vi "command engine process responses.vi"(8 "error out":errorcluster, 9 "State Variables":T1, 10 "Parameters":T4 {"Compiled"."MetaData"."Refs"."Data Reference" format="%.0x"; "Compiled"."Triggers"."Chan Refs" format="%.0x"; "Compiled"."Statuses"."Refs" format="%.0x"; "Compiled"."Data"."Refs" format="%.0x"; "Compiled"."Periodic Enable"."Refs"."Data Reference" format="%.0x"; "Compiled"."Wait Values"."Refs"."Data Reference" format="%.0x"; "Compiled"."External Channels"."Channels" format="%.0x"; "Compiled"."External Channels"."Triggers" format="%.0x"}, 11 "Global Variables":T17) -> (0 "error out":errorcluster, 1 "State Variables out":T1, 2 "Parameters out":T4 {"Compiled"."MetaData"."Refs"."Data Reference" format="%.0x"; "Compiled"."Triggers"."Chan Refs" format="%.0x"; "Compiled"."Statuses"."Refs" format="%.0x"; "Compiled"."Data"."Refs" format="%.0x"; "Compiled"."Periodic Enable"."Refs"."Data Reference" format="%.0x"; "Compiled"."Wait Values"."Refs"."Data Reference" format="%.0x"; "Compiled"."External Channels"."Channels" format="%.0x"; "Compiled"."External Channels"."Triggers" format="%.0x"}, 3 "Global Variables out":T17)   [LabVIEW 2013, in "Instrument Addon Engine.lvlib"]
uses:
  Instrument Addon Engine.lvlib
  Inline Async API/Controls/Engine State Variables.ctl
  Network Communication/TCP Refs.ctl
  Network Communication/Network Comm Global Ref.ctl
  Stop FG/Stop Global Ref.ctl
  <vilib>/NI/AMC/Message Queue.ctl
  <vilib>/NI/AMC/Message.ctl
  <vilib>/NI/Tools/Keyed Array/KeyedArray.ctl
  Types/Commands RT Configuration Cluster.ctl
  Protocols.lvlibp/Protocol Parent/Protocol Parent.lvclass
  Shared/Types/Compiled Settings.ctl
  Shared/Types/Command Parameters.ctl
  Shared/Types/Linked Channel Cluster.ctl
  <vilib>/NI Veristand/Custom Device API/Block Data Reference.ctl
  <vilib>/NI Veristand/Custom Device API/Data Reference.ctl
  Shared/Types/Response RT Configuration Cluster.ctl
  Shared/Types/Response Parameters.ctl
  Shared/Types/Response Wait Type.ctl
  Shared/Types/Message Parameters.ctl
  Shared/Types/Message Generation Type.ctl
  Shared/Types/External Trigger Refs.ctl
  Types/FIFO References.ctl
  Protections.lvlibp/Parent Protection/Protection.lvclass
  command engine global variables.ctl
  Stop FG/Stop FG.lvlib
  Network Communication/Network Common API.lvlib
  <vilib>/NI/Tools/Keyed Array/Tools_KeyedArray.lvlib
  <vilib>/NI/AMC/AMC.lvlib
  Inline Async API/Inline Async API.lvlib
  Shared/Instrument Addon Shared.lvlib
  <vilib>/NI Veristand/Custom Device API/Custom Device API.lvlib
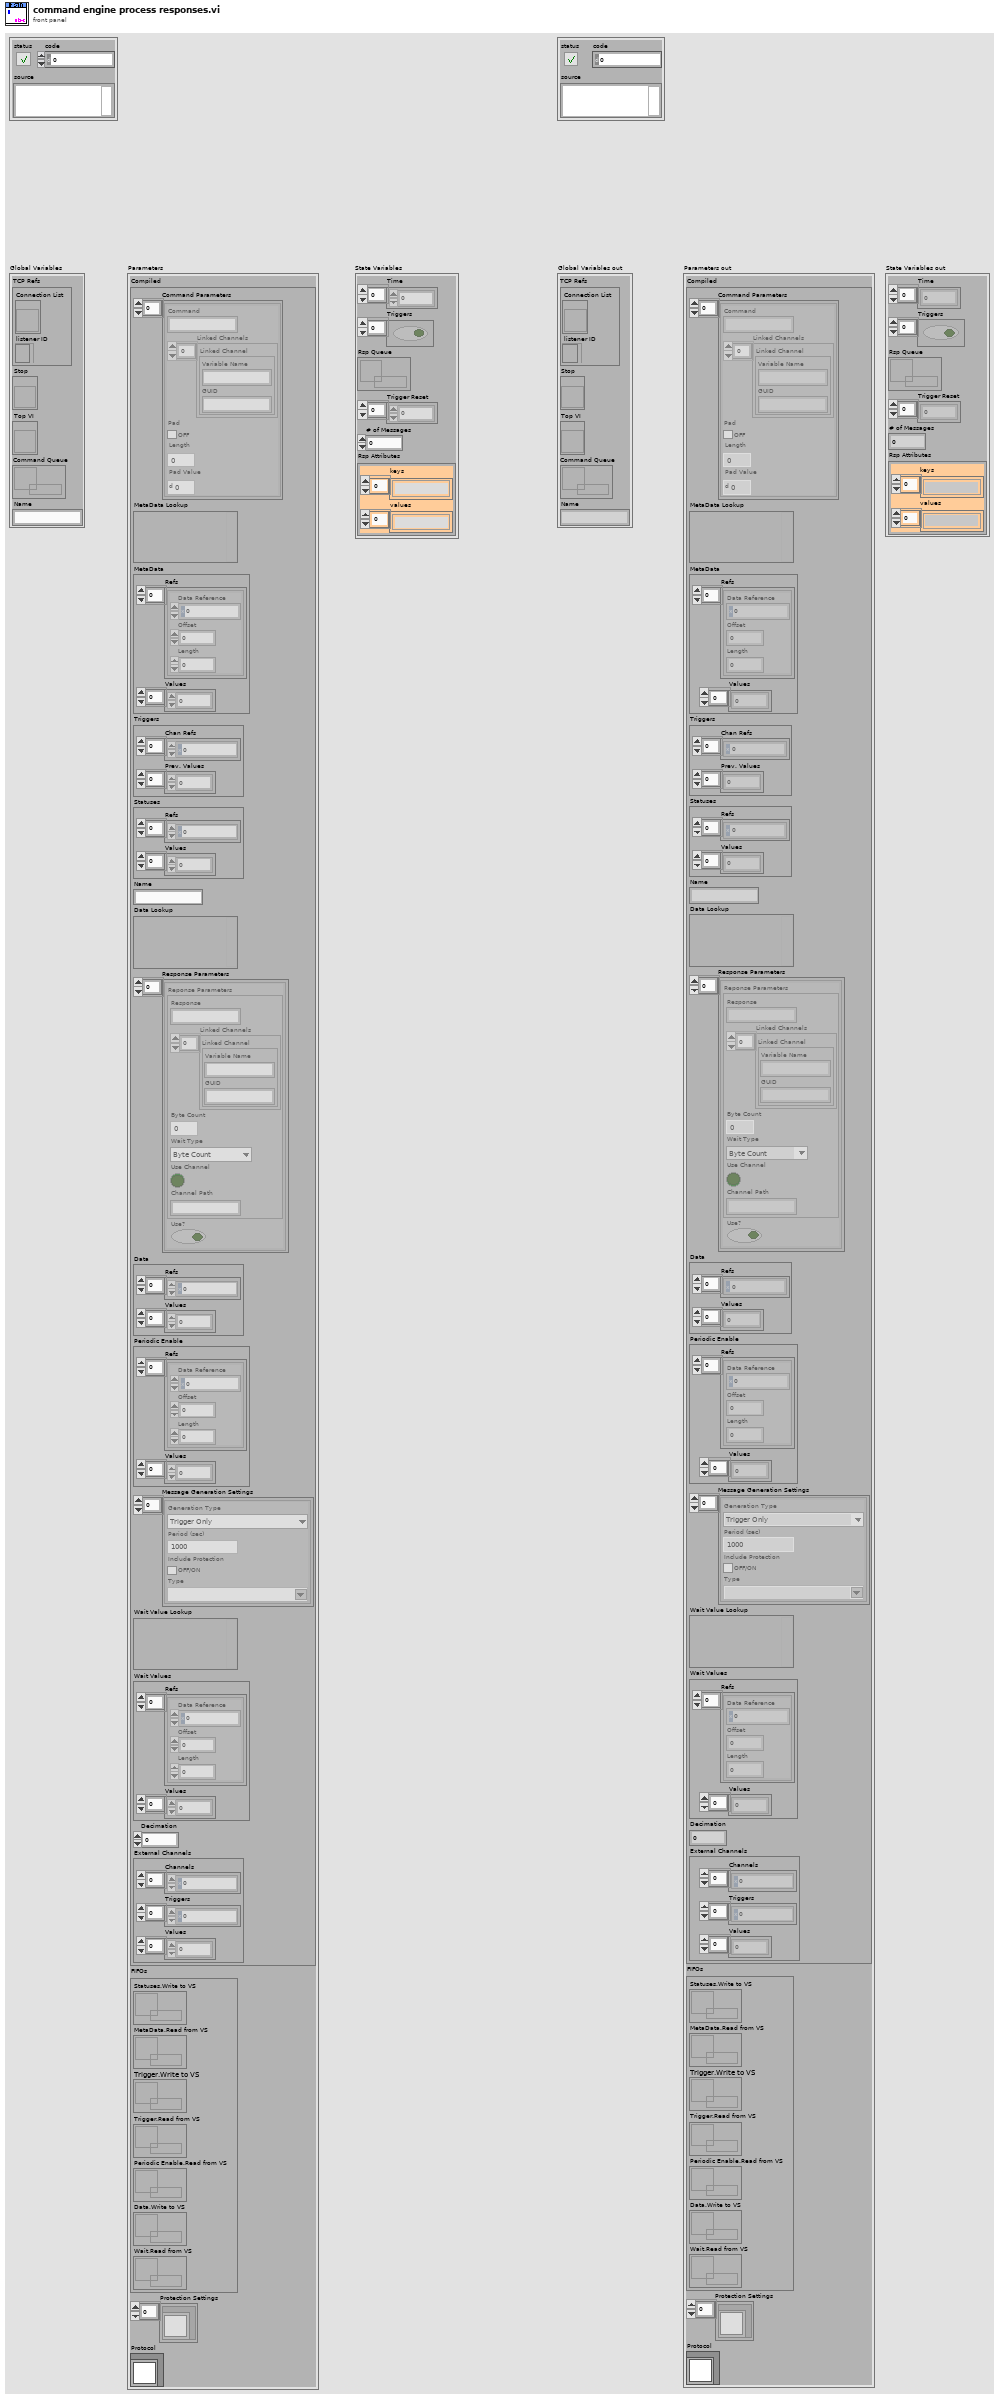
[diagram p1: front panel]
types:
  T1 = typedef "Instrument Addon Engine.lvlib/command engine global variables.ctl" = cluster{"Time":u32[], "Triggers":bool[], "Rsp Queue":T2, "Trigger Reset":dbl[], "# of Messages":i32, "Rsp Attributes":T3}
  T2 = typedef "AMC.lvlib/Message Queue.ctl" = refnum<queue>
  T3 = typedef "Tools_KeyedArray.lvlib/KeyedArray.ctl" = cluster{"keys":string[], "values":string[]}
  T4 = typedef "Instrument Addon Engine.lvlib/Commands RT Configuration Cluster.ctl" = cluster{"Compiled":T5, "FIFOs":T16, "Protection Settings":refnum<class "Protection.lvclass">[], "Protocol":refnum<class "Protocol Parent.lvclass">}
  T5 = typedef "Instrument Addon Shared.lvlib/Compiled Settings.ctl" = cluster{"Command Parameters":T6[], "MetaData Lookup":variant, "MetaData":cluster{"Refs":T8[], "Values":dbl[]}, "Triggers":cluster{"Chan Refs":T9[], "Prev. Values":dbl[]}, "Statuses":cluster{"Refs":T9[], "Values":dbl[]}, "Name":string, "Data Lookup":variant, "Response Parameters":T10[], "Data":cluster{"Refs":T9[], "Values":dbl[]}, "Periodic Enable":cluster{"Refs":T8[], "Values":dbl[]}, "Message Generation Settings":T13[], "Wait Value Lookup":variant, "Wait Values":cluster{"Refs":T8[], "Values":dbl[]}, "Decimation":u32, "External Channels":T15}
  T6 = typedef "Instrument Addon Shared.lvlib/Command Parameters.ctl" = cluster{"Command":string, "Linked Channels":T7[], "Pad":bool, "Length":u32, "Pad Value":u8}
  T7 = typedef "Instrument Addon Shared.lvlib/Linked Channel Cluster.ctl" = cluster{"Variable Name":string, "GUID":string}
  T8 = typedef "Custom Device API.lvlib/Block Data Reference.ctl" = cluster{"Data Reference":T9, "Offset":i32, "Length":i32}
  T9 = typedef "Custom Device API.lvlib/Data Reference.ctl" = i32
  T10 = typedef "Instrument Addon Shared.lvlib/Response RT Configuration Cluster.ctl" = cluster{"Reponse Parameters":T11, "Use?":bool}
  T11 = typedef "Instrument Addon Shared.lvlib/Response Parameters.ctl" = cluster{"Response":string, "Linked Channels":T7[], "Type Value":dbl, "Wait Type":T12, "Use Channel":bool, "Channel Path":string}
  T12 = typedef "Instrument Addon Shared.lvlib/Response Wait Type.ctl" = enum16{"Byte Count", "Wait sec"}
  T13 = typedef "Instrument Addon Shared.lvlib/Message Parameters.ctl" = cluster{"Generation Type":T14, "Period":dbl, "Include Protection":bool, "Type":string}
  T14 = typedef "Instrument Addon Shared.lvlib/Message Generation Type.ctl" = enum16{"Trigger Only", "Periodic & Trigger"}
  T15 = typedef "Instrument Addon Shared.lvlib/External Trigger Refs.ctl" = cluster{"Channels":T9[], "Triggers":T9[], "Values":dbl[]}
  T16 = typedef "Instrument Addon Engine.lvlib/FIFO References.ctl" = cluster{"Statuses.Write to VS":refnum<k33>, "MetaData.Read from VS":refnum<k33>, "Trigger.Write to VS":refnum<k33>, "Trigger.Read from VS":refnum<k33>, "Periodic Enable.Read from VS":refnum<k33>, "Data.Write to VS":refnum<k33>, "Wait.Read from VS":refnum<k33>}
  T17 = typedef "Instrument Addon Engine.lvlib/Inline Async API.lvlib/Engine State Variables.ctl" = cluster{"TCP Refs":T18, "Stop":T20, "Top VI":refnum<vi>, "Command Queue":T2, "Name":string}
  T18 = typedef "Instrument Addon Engine.lvlib/Network Common API.lvlib/TCP Refs.ctl" = cluster{"Connection List":T19, "listener ID":refnum<k5>}
  T19 = typedef "Instrument Addon Engine.lvlib/Network Common API.lvlib/Network Comm Global Ref.ctl" = refnum<vi>
  T20 = typedef "Instrument Addon Engine.lvlib/Stop FG.lvlib/Stop Global Ref.ctl" = refnum<vi>
  T21 = typedef "Instrument Addon Engine.lvlib/Buffered RT Instrument Request.ctl" = cluster{"Response":string, "Error":errorcluster}
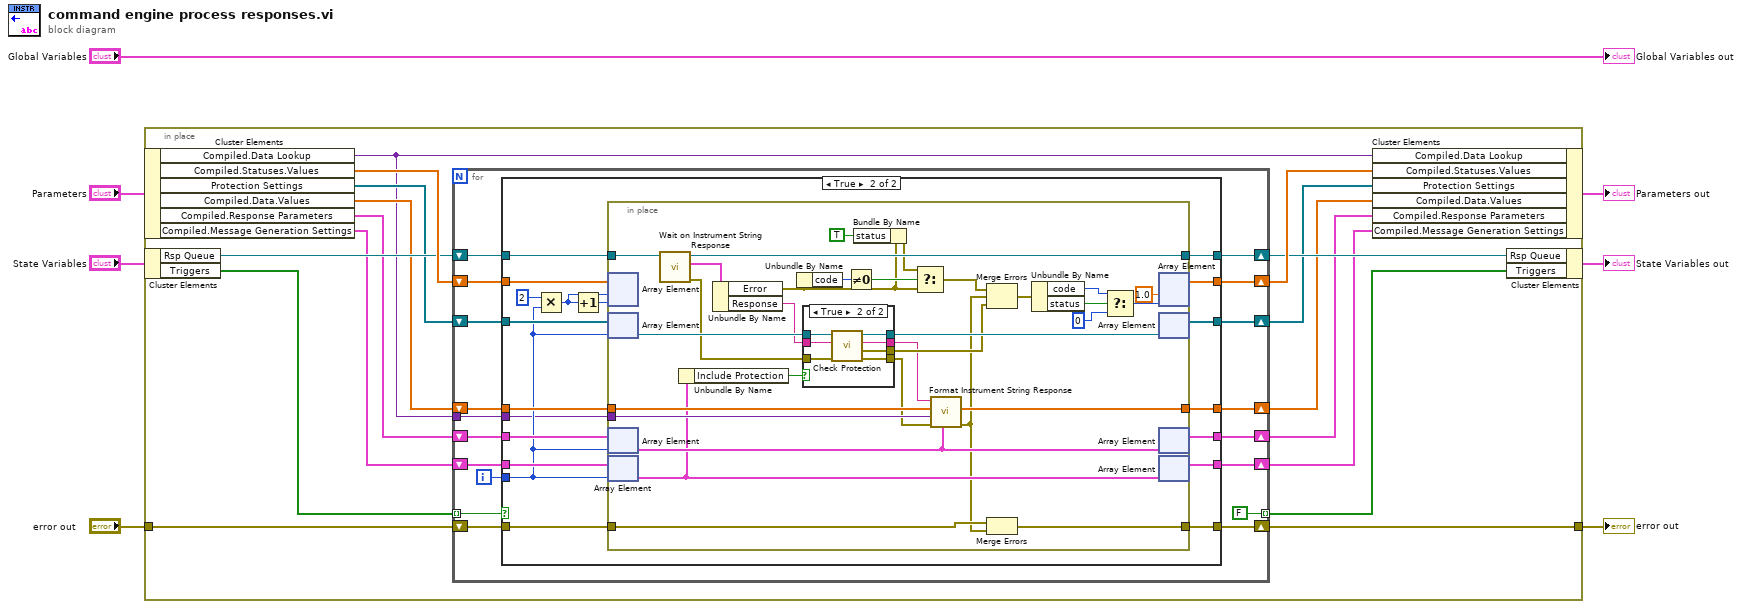
[diagram p0: block diagram]
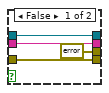
[diagram p3: hidden frame]
diagram:
  n1 = in-place {
    in-place-border: "error out" -> [w24]
    in-place-border: [w23] -> w7
    n2 = in-place-cluster #1("Parameters") -> ("Compiled.Data Lookup"=w8:variant, "Compiled.Statuses.Values"=w22:dbl[], "Protection Settings"=w10:refnum<class "Protection.lvclass">[], "Compiled.Data.Values"=w16:dbl[], "Compiled.Response Parameters"=w14:T10[], "Compiled.Message Generation Settings"=w13:T13[])
    n3 = in-place-cluster #2("State Variables") -> ("Rsp Queue"=w21:T2, "Triggers"=w20:bool[])
    n4 = for {
      shift-right: [w32] -> w19
      shift-left: w22 -> [w33]
      shift-right: [w42] -> w15
      shift-left: w16 -> [w40]
      shift-right: [w31] -> w9
      shift-left: w10 -> [w34]
      shift-right: [w27] -> w18
      shift-left: w21 -> [w28]
      shift-right: [w37] -> w11
      shift-left: w14 -> [w38]
      shift-right: [w35] -> w12
      shift-left: w13 -> [w36]
      tunnel: w8 -> [w29]
      shift-right: [w39] -> w23
      shift-left: w24 -> [w41]
      tunnel: w20 -> [w26] mode=indexing
      tunnel: [FALSE] -> w17 mode=indexing
      i -> [w30]
      n5 = case shown="True" w26 {
        tunnel: [w45 w68] -> w42
        tunnel: w41 -> [w46 w67]
        tunnel: w40 -> [w45 w66]
        tunnel: [w46 w65] -> w39
        tunnel: w38 -> [w44 w64]
        tunnel: [w44 w63] -> w37
        tunnel: w36 -> [w43 w62]
        tunnel: [w43 w61] -> w35
        tunnel: w34 -> [w49 w60]
        tunnel: w33 -> [w48 w59]
        tunnel: [w48 w55] -> w32
        tunnel: [w49 w54] -> w31
        tunnel: w30 -> [_ w53]
        tunnel: w29 -> [_ w52]
        tunnel: w28 -> [w47 w51]
        tunnel: [w47 w50] -> w27
        frame False {
        }
        frame True {
          n6 = Multiply(x=2, y=w53) -> (x*y=w57:i32)
          n7 = Increment(x=w57) -> (x+1=w56:i32)
          n8 = in-place {
            in-place-border: [w99] -> w68
            in-place-border: w67 -> [w98]
            in-place-border: w66 -> [w97]
            in-place-border: w52 -> [w96]
            in-place-border: [w95] -> w65
            in-place-border: w51 -> [w80]
            in-place-border: [w79] -> w50
            n9 = in-place-array #3(w59, w57, w56) -> ()  [unwired: 2 out]
            n10 = in-place-array #4(w60, w53) -> (w92:refnum<class "Protection.lvclass">)
            n11 = in-place-array #5(w64, w53) -> (w94:T10)
            n12 = in-place-array #6(w62, w53) -> (w93:T13)
            n13 = call "Wait on Instrument String Response.vi"("Response Queue"=w80) -> ("error out"=w88:errorcluster, "Response"=w81:T21, "message queue out"=w79:T2)  [unwired: 8 in]
            n14 = Unbundle By Name(w93) -> ("Include Protection"=w85:bool)
            n15 = Unbundle By Name(w81) -> ("Error"=w75:errorcluster, "Response"=w84:string)
            n16 = Unbundle By Name(w75) -> ("code"=w78:i32)
            n17 = case shown="True" w85 {
              tunnel: w88 -> [w102 w110]
              tunnel: w84 -> [w103 w109]
              tunnel: [w103 w107] -> w83
              tunnel: [errorcluster {"status"=FALSE, "code"=0, "source"=""} ("error out") w105] -> w87
              tunnel: [w102 w106] -> w86
              tunnel: w92 -> [w100 w108]
              tunnel: [w100 w104] -> w90
              frame False {
              }
              frame True {
                n18 = call-dynamic "Check Protection.vi"("error in (no error)"=w110, "String in"=w109, "Protection in"=w108) -> ("error out"=w106:errorcluster, "Protection Error"=w105:errorcluster, "String out"=w107:string, "Protection out"=w104:refnum<class "Protection.lvclass">)  [unwired: 5 in]
              }
            }
            n19 = Not Equal To 0?(x=w78) -> (x != 0?=w77:bool)
            n20 = Bundle By Name(cluster=w75, "status"=TRUE) -> (w74:errorcluster)
            n21 = Select(t=w74, s=w77, f=w75) -> (s? t:f=w76:errorcluster)
            n22 = call "Format Instrument String Response.vi"("Response Parameters"=w94, "error in (no error)"=w86, "Data Lookup in"=w96, "Data"=w97, "Response"=w83) -> ("error out"=w82:errorcluster, "Data out"=w99:dbl[])  [unwired: 4 in, 1 out]
            n23 = Merge Errors(w76, w82, w87) -> (w89:errorcluster)
            n24 = Merge Errors(w98, w82) -> (w95:errorcluster)
            n25 = Unbundle By Name(w89) -> ("code"=w70:i32, "status"=w72:bool)
            n26 = Select(t=w70, s=w72, f=0) -> (s? t:f=w71:i32)
            n27 = in-place-array #3(1.0, w71) -> (w55:dbl[])  [unwired: 2 out]
            n28 = in-place-array #4(w90) -> (w54:refnum<class "Protection.lvclass">[])  [unwired: 1 out]
            n29 = in-place-array #5(w94) -> (w63:T10[])  [unwired: 1 out]
            n30 = in-place-array #6(w93) -> (w61:T13[])  [unwired: 1 out]
          }
        }
      }
    }
    n31 = in-place-cluster #1("Compiled.Data Lookup"=w8, "Compiled.Statuses.Values"=w19, "Protection Settings"=w9, "Compiled.Data.Values"=w15, "Compiled.Response Parameters"=w11, "Compiled.Message Generation Settings"=w12) -> (→"Parameters out":T4)
    n32 = in-place-cluster #2("Rsp Queue"=w18, "Triggers"=w17) -> (→"State Variables out":T1)
  }
  "error out" <- w7
  "Global Variables out" <- "Global Variables"
